vi "Test 7.vi"(8 "error in (no error)":errorcluster, 11 "Test Case In":refnum<class "Tests.lvclass">) -> (0 "error out":errorcluster, 3 "Test Case Out":refnum<class "Tests.lvclass">)   [LabVIEW 2020, in "Tests.lvclass"]
uses:
  Tests.lvclass
  Tests.lvclass/Tests.ctl
  Proto/NetAn.lvclass
  <vilib>/Astemes/LUnit/Test Case.lvclass
  C:/Program Files (x86)/National Instruments/LabVIEW 2020/vi.lib/Astemes/LUnit/Test Case.lvclass
  C:/Program Files (x86)/National Instruments/LabVIEW 2020/vi.lib/Astemes/LUnit/LUnit Runnable.lvclass
  C:/git/aoc-2024/Day 23/Tests/Tests.lvclass
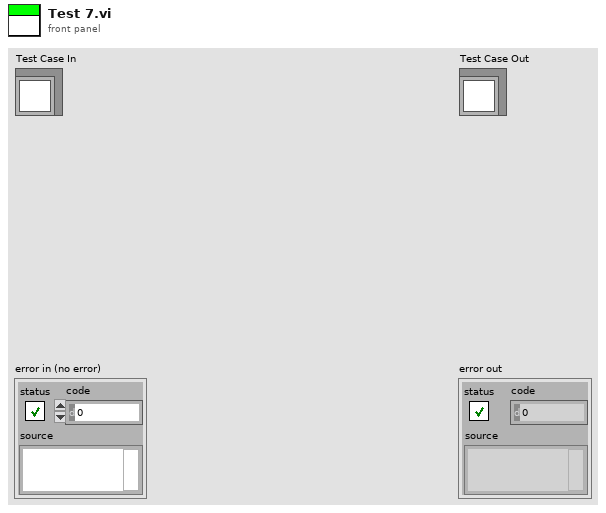
[diagram p1: front panel]
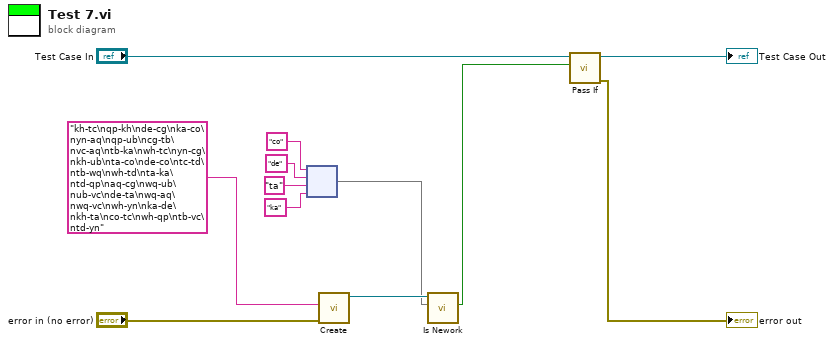
[diagram p0: block diagram]
diagram:
  n1 = node("co" ("element"), "de" ("element"), "ta" ("element"), "ka" ("element")) -> (w3:set{string})
  n2 = call "Create.vi"("error in (no error)"="error in (no error)", "Input"="kh-tc\nqp-kh\nde-cg\nka-co\nyn-aq\nqp-ub\ncg-tb\nvc-aq\ntb-ka\nwh-tc\nyn-cg\nkh-ub\nta-co\nde-co\ntc-td\ntb-wq\nwh-td\nta-ka\ntd-qp\naq-cg\nwq-ub\nub-vc\nde-ta\nwq-aq\nwq-vc\nwh-yn\nka-de\nkh-ta\nco-tc\nwh-qp\ntb-vc\ntd-yn") -> ("Proto"=w8:refnum<class "NetAn.lvclass">)  [unwired: 8 in, 1 out]
  n3 = call "Is Nework.vi"("Set"=w3, "NetAn in"=w8) -> ("Is network"=w2:bool)  [unwired: 8 in, 1 out]
  n4 = call <vilib>:"Pass If.vi"("Pass?"=w2, "LUnit Test Case In"="Test Case In") -> ("error out"=→"error out":errorcluster, "LUnit Test Case Out"=→"Test Case Out":refnum<class "Tests.lvclass">)  [unwired: 8 in]
